vi "MEScope_SetPower.vi"(8 "error in (no error)":errorcluster, 11 "bPowerOnOff":i8) -> (0 "error out":errorcluster, 3 "return type":i32)   [LabVIEW 2015]
doc: "ScopeSetPower\n\nDescription: \nCall this function to power on/off the DSP section via the Cypress chip.\nDetail: \nint ScopeSetPower (\nBYTE bPowerOnOff\n); \n\nParameters:\nBYTE bPowerOnOff - Byte Value set to 1 to turn on power and 0 to turn off.\n\nReturn Values:\nA returned value of 0 indicates success. A non-zero return code will indicate error."
uses:
  ScannerDiagDLL.dll
panel:
  # "Value set to 1 to turn on power and 0 to turn off"
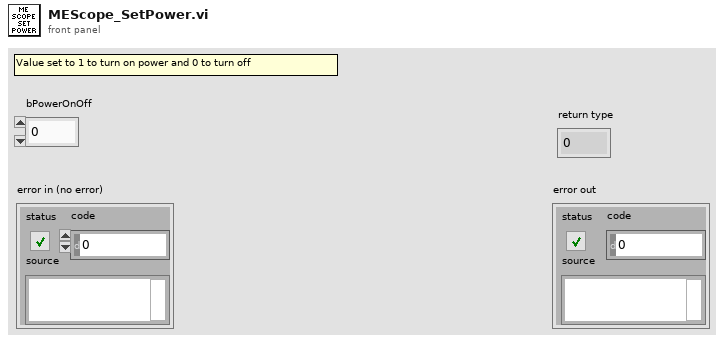
[diagram p1: front panel]
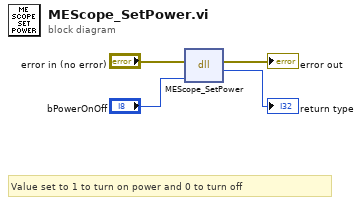
[diagram p0: block diagram]
diagram:
  # "Value set to 1 to turn on power and 0 to turn off"
  n1 = dll-call lib="C:/ModisEdge/Scope/Test Sequence/Code Modules/DLL/ScannerDiagDLL.dll" fn="MEScope_SetPower"(error in="error in (no error)", "arg1"="bPowerOnOff") -> (error out=→"error out":errorcluster, "return type"=→"return type":i32)  [unwired: 3 in, 1 out]
